vi "Pelletron_Monitor.vi"() -> ()   [LabVIEW 2009, in "AccelNET.lvlib" / "Control_VIs.lvlib"]
uses:
  Control_VIs.lvlib
  Component_Power_Indicator.ctl
  Interlocks.ctl
  Parameters_Indicator.ctl
  Bypass_Indicator.ctl
  TCPinfo.vi
  TCP.lvclass
  Global_Variables.lvlib
  Useful_SubVIs.lvlib
  Useful_Controls.lvlib
panel:
  in  "Clear Errors":bool
  out "Parameters":T1 {"Lost Charge (uA)" scale=-10.0..10.0; "Radiation (mRad/hr)" step=3.978696e-316 scale=0.02..200.0; "Vacuum (Torr)" scale=1e-09..0.001 scale format="%#_6e"}
  out "Interlock Status":T2
  out "Pelletron Bypass":T3
  out "Component\nPower":T4
  out "Queue Error":errorcluster
  out "Accelnet Errors":errorcluster
  in  "stop":bool
  out "Start Time":dbl format="%<%m/%d/%Y  -  %H:%M:%S>T"
  in  "Clear":bool
  in  "X Maximum":dbl max=0.0 step=30.0 format="%<%H:%M:%S>t"
  in  "X Autoscale":bool=TRUE
  in  "X Minimum":dbl max=0.0 step=30.0 format="%<%H:%M:%S>t"
  in  "Y Autoscale":bool=TRUE
  in  "Y Maximum":dbl
  in  "Y Minimum":dbl
  out "XY Graph":cluster{dbl[], dbl[]}(graph)
  in  "Plotter\nSelector":u16(ring) items=["High Voltage", "High Voltage PS", "Chain Current", "Column Current", "Lost Charge", "Radiation", "Pressure", "HV Control Difference"]
  # "Controls"
  # "Parameters"
  # "Interlocks"
  # "Bypass"
  # "Component On/Off"
  # "Pelletron Plotter"
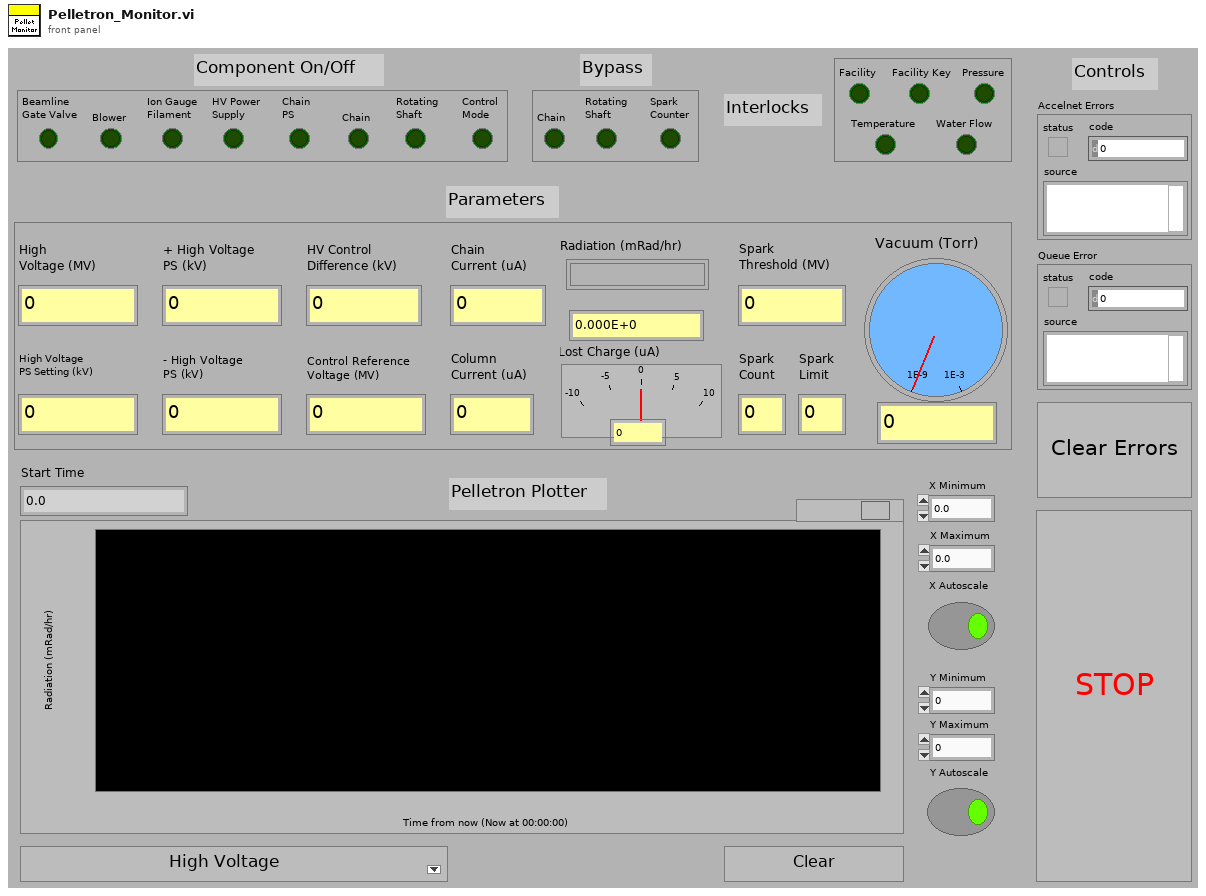
[diagram p1: front panel]
types:
  T1 = typedef "AccelNET.lvlib/Useful_Controls.lvlib/Parameters_Indicator.ctl" = cluster{"Vacuum (Torr)":dbl, "Radiation (mRad/hr)":dbl, "Spark\nThreshold (MV)":dbl, "Lost Charge (uA)":dbl, "Spark\nCount":dbl, "Spark\nLimit":dbl, "Column\nCurrent (uA)":dbl, "Chain\nCurrent (uA)":dbl, "High Voltage\nPS Setting (kV)":dbl, "HV Control\nDifference (kV)":dbl, "- High Voltage\nPS (kV)":dbl, "+ High Voltage\nPS (kV)":dbl, "Control Reference\nVoltage (MV)":dbl, "High\nVoltage (MV)":dbl}
  T2 = typedef "AccelNET.lvlib/Useful_Controls.lvlib/Interlocks.ctl" = cluster{"Facility":bool, "Facility Key":bool, "Water Flow":bool, "Pressure":bool, "Temperature":bool}
  T3 = typedef "AccelNET.lvlib/Useful_Controls.lvlib/Bypass_Indicator.ctl" = cluster{"Chain":bool, "Rotating\nShaft":bool, "Spark\nCounter":bool}
  T4 = typedef "AccelNET.lvlib/Useful_Controls.lvlib/Component_Power_Indicator.ctl" = cluster{"Beamline\nGate Valve":bool, "Blower":bool, "Chain":bool, "Rotating\nShaft":bool, "HV Power\nSupply":bool, "Ion Gauge\nFilament":bool, "Control\nMode":bool, "Chain\nPS":bool}
  T5 = cluster{"Time":dbl, "High Voltage":dbl, "High VoltagePS":dbl, "Chain Current":dbl, "Column Current":dbl, "Lost Charge":dbl, "Radiation":dbl, "Pressure":dbl, "HV Control Difference":dbl}[]
  T6 = cluster{"Timestamp":u64, "High Voltage":sgl, "Vacuum Pressure":sgl, "Column Current":sgl, "Chain Current":sgl, "- High Voltage Supply":dbl, "+ High Voltage Supply":dbl, "Radiation":dbl, "Lost Charge":dbl, "Control High Voltage":dbl, "HV Control Difference":dbl}
  T7 = cluster{"Time":dbl, "High Voltage":dbl, "High VoltagePS":dbl, "Chain Current":dbl, "Column Current":dbl, "Lost Charge":dbl, "Radiation":dbl, "Pressure":dbl, "HV Control Difference":dbl}
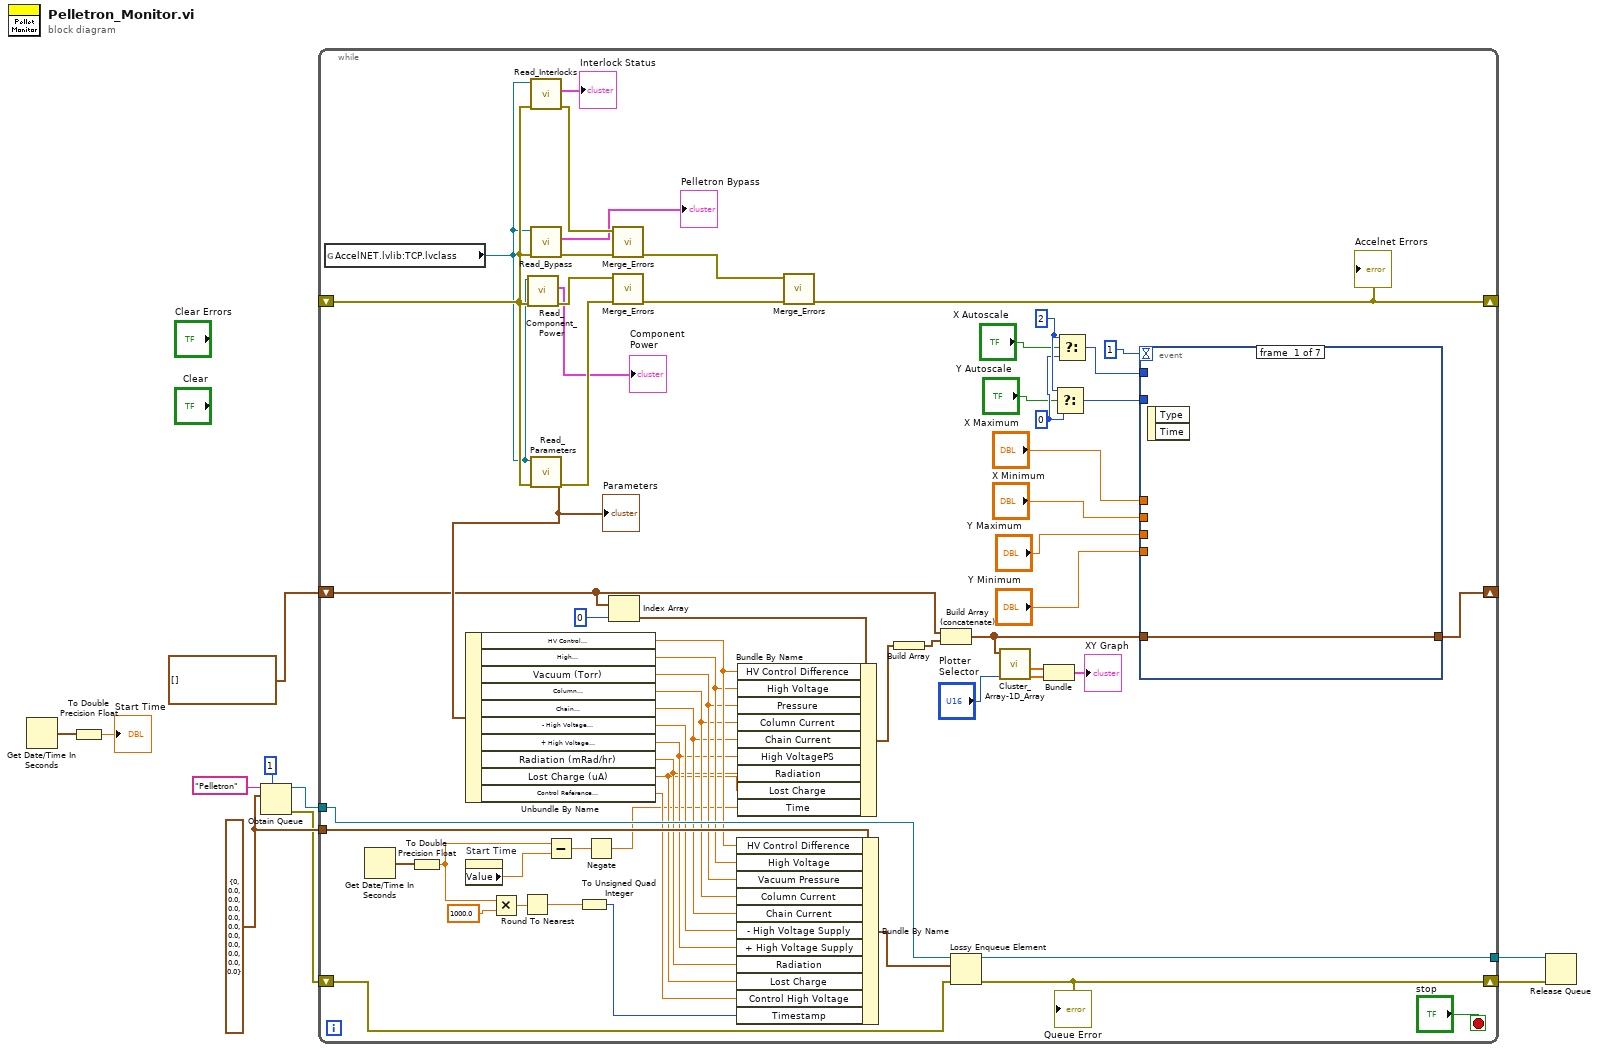
[diagram p0: block diagram]
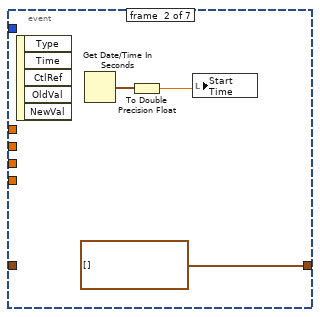
[diagram p2: hidden frame]
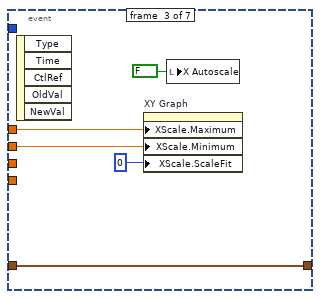
[diagram p3: hidden frame]
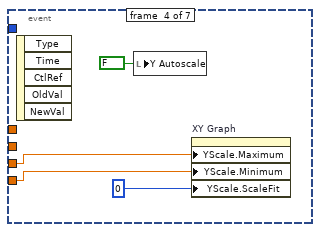
[diagram p4: hidden frame]
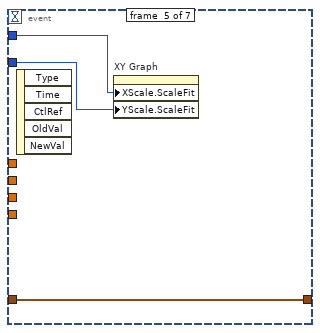
[diagram p5: hidden frame]
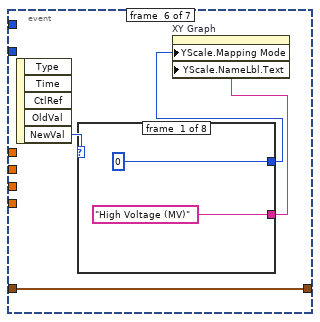
[diagram p6: hidden frame]
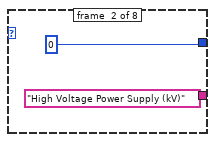
[diagram p7: hidden frame]
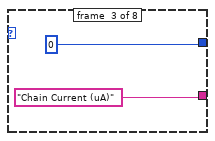
[diagram p8: hidden frame]
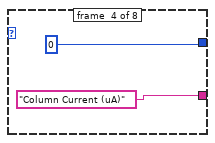
[diagram p9: hidden frame]
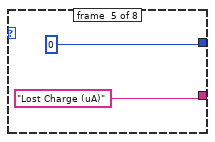
[diagram p10: hidden frame]
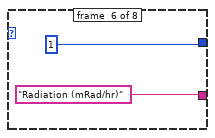
[diagram p11: hidden frame]
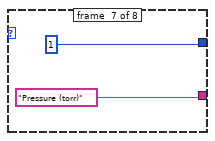
[diagram p12: hidden frame]
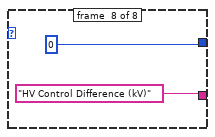
[diagram p13: hidden frame]
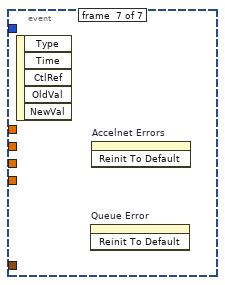
[diagram p14: hidden frame]
diagram:
  w5 = T6 {"Timestamp"=0, "High Voltage"=0.0, "Vacuum Pressure"=0.0, "Column Current"=0.0, "Chain Current"=0.0, "- High Voltage Supply"=0.0, "+ High Voltage Supply"=0.0, "Radiation"=0.0, "Lost Charge"=0.0, "Control High Voltage"=0.0, "HV Control Difference"=0.0} ("Cluster")
  n1 = Get Date/Time In Seconds() -> (seconds since 1Jan1904=w9:timestamp)
  n2 = To Double Precision Float(number=w9) -> (double precision float=→"Start Time":dbl)
  n3 = Obtain Queue(max queue size (-1, unlimited)=1, name (unnamed)="Pelletron", element data type=w5) -> (queue out=w4:refnum<queue>, error out=w3:errorcluster)  [unwired: 2 in, 1 out]
  n4 = while {
    shift-right: [w63] -> _
    shift-left: _ -> [w70]
    shift-right: [w39] -> _
    shift-left: T5 [] -> [w27]
    tunnel: w5 -> [w35]
    tunnel: w4 -> [w34]
    shift-right: [w32] -> w1
    shift-left: w3 -> [w31]
    tunnel: [w33] -> w2
    stop <- "stop" stop-if-true
    w53 = 0
    w54 = 2
    n5 = global read "TCPinfo.vi" "AccelNET.lvlib:TCP.lvclass"() -> (w49:refnum<class "TCP.lvclass">)
    n6 = Get Date/Time In Seconds() -> (seconds since 1Jan1904=w62:timestamp)
    n7 = To Double Precision Float(number=w62) -> (double precision float=w48:dbl)
    n8 = property on="Start Time" class="DigNum (strict)"() -> ("Value"=w61:dbl)  [unwired: 2 in, 2 out]
    n9 = Multiply(x=w48, y=1000.0) -> (x*y=w46:dbl)
    n10 = Round To Nearest(number=w46) -> (nearest integer value=w41:dbl)
    n11 = call "Read_Component_Power.vi"("error in (no error)"=w70, "AccelNET.lvlib:TCP.lvclass"=w49) -> ("Error Out"=w67:errorcluster, "Component Power"=→"Component\nPower":T4)  [unwired: 8 in]
    n12 = call "Read_Interlocks.vi"("Error In"=w70, "AccelNET.lvlib:TCP.lvclass"=w49) -> ("Error Out"=w69:errorcluster, "Interlock Status"=→"Interlock Status":T2)  [unwired: 8 in]
    n13 = call "Read_Bypass.vi"("error in (no error)"=w70, "AccelNET.lvlib:TCP.lvclass"=w49) -> ("Error Out"=w68:errorcluster, "Pelletron Bypass"=→"Pelletron Bypass":T3)  [unwired: 8 in]
    n14 = call "Read_Parameters.vi"("error in (no error)"=w70, "AccelNET.lvlib:TCP.lvclass"=w49) -> ("Error Out"=w66:errorcluster, "Parameters"=w50:T1)  [unwired: 8 in]
    "Parameters" <- w50
    n15 = Unbundle By Name(w50) -> ("HV Control\nDifference (kV)"=w23:dbl, "High\nVoltage (MV)"=w22:dbl, "Vacuum (Torr)"=w21:dbl, "Column\nCurrent (uA)"=w20:dbl, "Chain\nCurrent (uA)"=w19:dbl, "- High Voltage\nPS (kV)"=w25:dbl, "+ High Voltage\nPS (kV)"=w18:dbl, "Radiation (mRad/hr)"=w17:dbl, "Lost Charge (uA)"=w16:dbl, "Control Reference\nVoltage (MV)"=w24:dbl)
    n16 = Subtract(x=w48, y=w61) -> (x-y=w29:dbl)
    n17 = To Unsigned Quad Integer(1:w41) -> (0:w26:u64)
    n18 = Negate(x=w29) -> (-x=w15:dbl)
    n19 = Index Array(array=w27, index=0) -> (element=w36:T7)
    n20 = call "Merge_Errors.vi"("Error 2"=w68, "Error 1"=w69) -> ("Error Out"=w65:errorcluster)  [unwired: 9 in]
    n21 = call "Merge_Errors.vi"("Error 2"=w66, "Error 1"=w67) -> ("Error Out"=w64:errorcluster)  [unwired: 9 in]
    n22 = Bundle By Name(cluster=w35, "HV Control Difference"=w23, "High Voltage"=w22, "Vacuum Pressure"=w21, "Column Current"=w20, "Chain Current"=w19, "- High Voltage Supply"=w25, "+ High Voltage Supply"=w18, "Radiation"=w17, "Lost Charge"=w16, "Control High Voltage"=w24, "Timestamp"=w26) -> (w38:T6)
    n23 = Bundle By Name(cluster=w36, "HV Control Difference"=w23, "High Voltage"=w22, "Pressure"=w21, "Column Current"=w20, "Chain Current"=w19, "High VoltagePS"=w18, "Radiation"=w17, "Lost Charge"=w16, "Time"=w15) -> (w40:T7)
    n24 = call "Merge_Errors.vi"("Error 2"=w64, "Error 1"=w65) -> ("Error Out"=w63:errorcluster)  [unwired: 9 in]
    "Accelnet Errors" <- w63
    n25 = Build Array(w40) -> (w28:T5)
    n26 = Build Array (concatenate)(w27, w28) -> (w30:T5)
    n27 = Lossy Enqueue Element(queue=w34, element=w38, error in (no error)=w31) -> (queue out=w33:refnum<queue>, error out=w32:errorcluster)  [unwired: 2 out]
    "Queue Error" <- w32
    n28 = call "Cluster_Array-1D_Array.vi"("Plotter Selector"="Plotter\nSelector", "Input Cluster"=w30) -> ("Output Data"=w44:dbl[], "Time"=w42:dbl[])  [unwired: 8 in]
    n29 = Bundle("Time"=w42, "Output Data"=w44) -> (→"XY Graph":cluster{"Time":dbl[], "Output Data":dbl[]})  [unwired: 1 in]
    n30 = Select(t=w54, s="Y Autoscale", f=w53) -> (s? t:f=w52:i32)
    n31 = Select(t=w54, s="X Autoscale", f=w53) -> (s? t:f=w51:i32)
    n32 = event shown="[3] \"Y Maximum\", \"Y Minimum\": Value Change" {
      selector: _ -> [_ _ _ _ _ _ _]
      dyn-events: _ -> [_ _ _ _ _ _ _]
      timeout: 1 -> [_ _ _ _ _ _ _]
      tunnel: "X Maximum" -> [_ _ w80 _ _ _ _]
      tunnel: "X Minimum" -> [_ _ w79 _ _ _ _]
      tunnel: "Y Maximum" -> [_ _ _ w81 _ _ _]
      tunnel: "Y Minimum" -> [_ _ _ w82 _ _ _]
      tunnel: w52 -> [_ _ _ _ w86 _ _]
      tunnel: w51 -> [_ _ _ _ w85 _ _]
      tunnel: w30 -> [w72 _ w76 _ w87 w91 _]
      tunnel: [w72 T5 [] w76 _ w87 w91 _] -> w39
      event #0 {
        n33 = event-data() -> ()  [unwired: 1 in, 2 out]
      }
      event #1 {
        n34 = event-data() -> ()  [unwired: 1 in, 5 out]
        n35 = Get Date/Time In Seconds() -> (seconds since 1Jan1904=w75:timestamp)
        n36 = To Double Precision Float(number=w75) -> (double precision float=w74:dbl)
        n37 = local write "Start Time"(w74) -> ()
      }
      event #2 {
        n38 = event-data() -> ()  [unwired: 1 in, 5 out]
        n39 = property on="XY Graph" class="XYGraph (strict)"("XScale.Maximum"=w80, "XScale.Minimum"=w79, "XScale.ScaleFit"=u8 0 ("X Scale.Scale Fit")) -> ()  [unwired: 2 in, 2 out]
        n40 = local write "X Autoscale"(FALSE ("X Autoscale")) -> ()
      }
      event #3 {
        n41 = event-data() -> ()  [unwired: 1 in, 5 out]
        n42 = local write "Y Autoscale"(FALSE ("Y Autoscale")) -> ()
        n43 = property on="XY Graph" class="XYGraph (strict)"("YScale.Maximum"=w81, "YScale.Minimum"=w82, "YScale.ScaleFit"=u8 0 ("X Scale.Scale Fit")) -> ()  [unwired: 2 in, 2 out]
      }
      event #4 {
        n44 = event-data() -> ()  [unwired: 1 in, 5 out]
        n45 = property on="XY Graph" class="XYGraph (strict)"("XScale.ScaleFit"=w85, "YScale.ScaleFit"=w86) -> ()  [unwired: 2 in, 2 out]
      }
      event #5 {
        n46 = event-data() -> ("NewVal"=w90:u16)  [unwired: 1 in, 4 out]
        n47 = case shown="3" w90 {
          tunnel: [0 0 0 0 0 1 1 0] -> w89
          tunnel: ["High Voltage (MV)" "High Voltage Power Supply (kV)" "Chain Current (uA)" "Column Current (uA)" "Lost Charge (uA)" "Radiation (mRad/hr)" "Pressure (torr)" "HV Control Difference (kV)"] -> w88
          frame #0 {
          }
          frame #1 {
          }
          frame #2 {
          }
          frame #3 {
          }
          frame #4 {
          }
          frame #5 {
          }
          frame #6 {
          }
          frame #7 {
          }
        }
        n48 = property on="XY Graph" class="XYGraph (strict)"("YScale.Mapping Mode"=w89, "YScale.NameLbl.Text"=w88) -> ()  [unwired: 2 in, 2 out]
      }
      event #6 {
        n49 = event-data() -> ()  [unwired: 1 in, 5 out]
        n50 = invoke on="Queue Error" class="Clust (strict)" method="Reinit To Default"() -> ()  [unwired: 3 in, 3 out]
        n51 = invoke on="Accelnet Errors" class="Clust (strict)" method="Reinit To Default"() -> ()  [unwired: 3 in, 3 out]
      }
    }
  }
  n52 = Release Queue(queue=w2, error in (no error)=w1) -> ()  [unwired: 1 in, 3 out]
